vi "Get popup location.vi"(10 "Coords":T3, 11 "D_Datagrid in":refnum<class "D_Datagrid.lvclass">) -> (0 "Cell Position":T1, 1 "In bounds?":bool, 2 "Valid cell?":bool, 3 "Bounds":T2)   [LabVIEW 2023, in "D Datagrid Library.lvlib" / "D_Datagrid.lvclass"]
uses:
  D_Datagrid.lvclass
  <vilib>/Utility/miscctls.llb/LVPoint32TypeDef.ctl
  <vilib>/Utility/miscctls.llb/LVRectTypeDef.ctl
  <vilib>/Utility/miscctls.llb/LVRowAndColumnTypeDef.ctl
  D_Datagrid.lvclass/D_Datagrid.ctl
  Read DataElements.vi
  DatagridElement/DatagridElement.lvclass
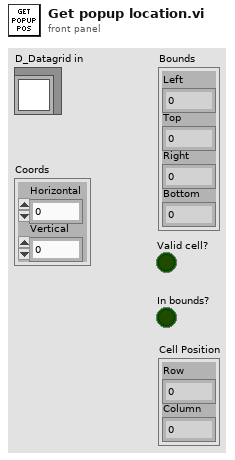
[diagram p1: front panel]
types:
  T1 = typedef "LVRowAndColumnTypeDef.ctl" = cluster{"Row":i32, "Column":i32}
  T2 = typedef "LVRectTypeDef.ctl" = cluster{"Left":i16, "Top":i16, "Right":i16, "Bottom":i16}
  T3 = typedef "LVPoint32TypeDef.ctl" = cluster{"Horizontal":i32, "Vertical":i32}
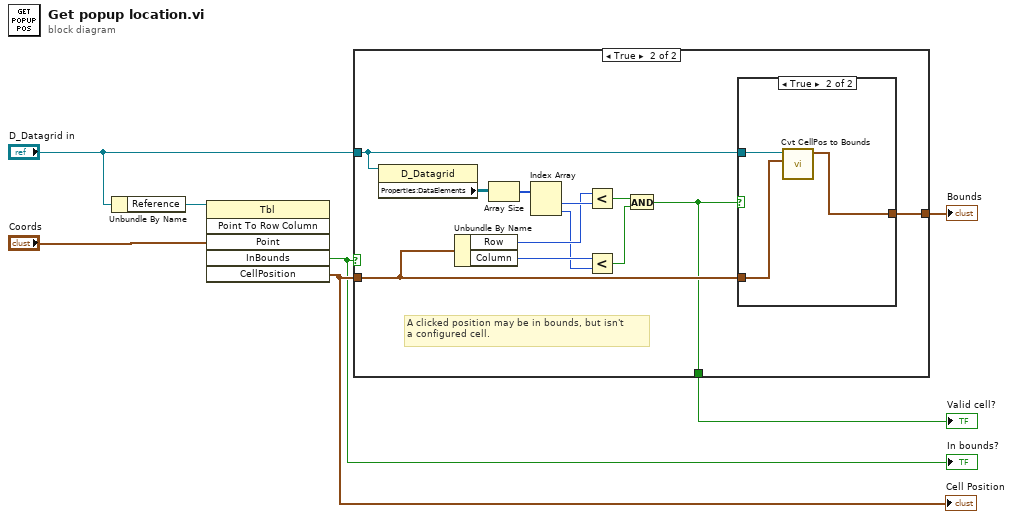
[diagram p0: block diagram]
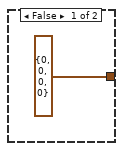
[diagram p3: hidden frame]
diagram:
  n1 = Unbundle By Name("D_Datagrid in") -> ("Reference"=w3:refnum<vi>)
  n2 = invoke class="Tbl" method="Point To Row Column"(reference=w3, "Point"="Coords") -> ("InBounds"=w2:bool, "CellPosition"=w5:T1)  [unwired: 4 in, 4 out]
  "In bounds?" <- w2
  "Cell Position" <- w5
  n3 = case shown="True" w2 {
    selector: w2 -> [w8 _]
    tunnel: "D_Datagrid in" -> [_ w19]
    tunnel: w5 -> [_ w17]
    tunnel: [_ w20] -> w4
    tunnel: [w8 w9] -> w1
    frame False {
    }
    frame True {
      # "A clicked position may be in bounds, but isn't\na configured cell."
      n4 = property class="D_Datagrid"(reference=w19) -> ("Properties:DataElements"=w18:refnum<class "DatagridElement.lvclass">[][])  [unwired: 1 in, 2 out]
      n5 = Unbundle By Name(w17) -> ("Row"=w14:i32, "Column"=w13:i32)
      n6 = Array Size(array=w18) -> (size(s)=w16:i32[])
      n7 = Index Array(array=w16) -> (element #1=w15:i32, element #2=w12:i32)  [unwired: 2 in]
      n8 = Less?(x=w14, y=w15) -> (x < y?=w11:bool)
      n9 = Less?(x=w13, y=w12) -> (x < y?=w10:bool)
      n10 = And(x=w11, y=w10) -> (x .and. y?=w9:bool)
      n11 = case shown="True" w9 {
        tunnel: w19 -> [_ w24]
        tunnel: w17 -> [_ w23]
        tunnel: [T2 {"Left"=0, "Top"=0, "Right"=0, "Bottom"=0} ("Bounds") w22] -> w20
        frame False {
        }
        frame True {
          n12 = call "Cvt CellPos to Bounds.vi"("CellPosition"=w23, "D_Datagrid in"=w24) -> ("Bounds"=w22:T2)  [unwired: 9 in]
        }
      }
    }
  }
  "Bounds" <- w4
  "Valid cell?" <- w1
